vi "调用main.vi"(1 "是否调用?":bool=TRUE) -> (0 "发生错误?":bool=TRUE)   [LabVIEW 2017]
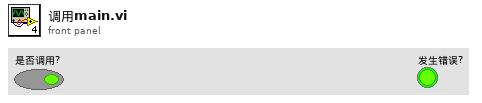
[diagram p1: front panel]
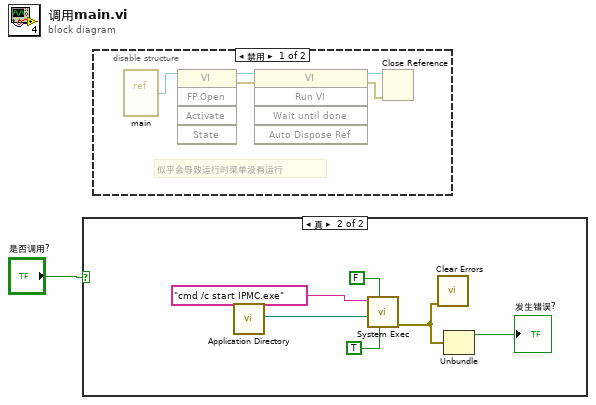
[diagram p0: block diagram]
diagram:
  n1 = case shown="真" "是否调用?" {
    frame False {
    }
    frame True {
      n2 = call <vilib>:"Application Directory.vi"() -> ("Application Directory"=w7:path)
      n3 = call <vilib>:"System Exec.vi"("run minimized? (F)"=TRUE, "wait until completion? (T)"=FALSE, "working directory"=w7, "command line"="cmd /c start IPMC.exe") -> ("error out"=w2:errorcluster)  [unwired: 4 in, 3 out]
      n4 = call <vilib>:"Clear Errors.vi"("error in (no error)"=w2) -> ()  [unwired: 5 in, 2 out]
      n5 = Unbundle(w2) -> ("status"=→"发生错误?":bool)  [unwired: 2 out]
    }
  }
  n6 = disable-structure shown="禁用" {
    frame Disabled {
      # "似乎会导致运行时菜单没有运行"
      n7 = vi-ref "main.vi"() -> (w12:refnum<vi>)
      n8 = invoke class="VI" method="FP.Open"(reference=w12) -> (reference out=w11:refnum<vi>, error out=w8:errorcluster)  [unwired: 4 in, 3 out]
      n9 = invoke class="VI" method="Run VI"(reference=w11, error in=w8) -> (reference out=w10:refnum<vi>, error out=w9:errorcluster)  [unwired: 3 in, 3 out]
      n10 = Close Reference(reference=w10, error in (no error)=w9) -> ()  [unwired: 1 out]
    }
    frame Enabled {
    }
  }
